vi "Pop-up wait prompt + events block.vi"(6 "Is Dialog?":enum16{"Normal", "Dialog Box"}(ring), 8 "error in (no error)":errorcluster, 9 "Prompt Text":string, 11 "Control":enum16{"Open", "Close", "Status", "No Change"}(ring)) -> (0 "error out":errorcluster)   [LabVIEW 2013]
doc: "If there is no error in, this vi will either open or close the calling panel which displays a prompt to wait. The input control determines whether the panel is opened or closed. Typically called before intensive processing with control=open and after with control = close.\n\nClose action ignores error in."
uses:
  GUI.lvlib
  Timing/Timing Lib.lvlib
panel:
  out "Prompt":string
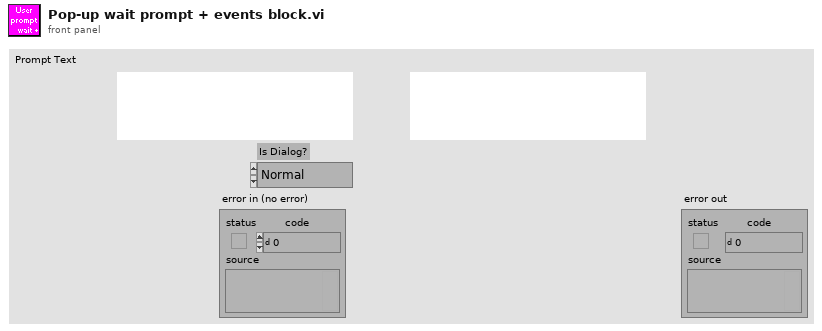
[diagram p1: front panel]
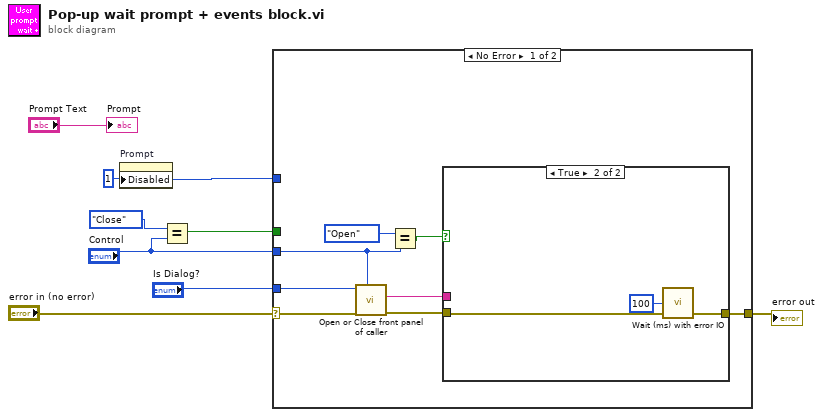
[diagram p0: block diagram]
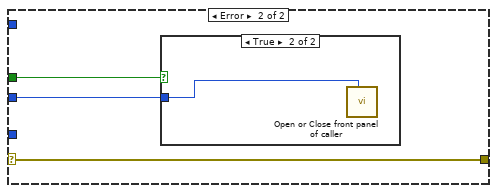
[diagram p3: hidden frame]
diagram:
  w4 = u8 1 ("Write Attribute")
  n1 = property on="Prompt" class="Str"("Disabled"=w4) -> ()  [unwired: 2 in, 2 out]
  n2 = Equal?(x=enum16{"Open", "Close", "Status", "No Change"}."Close", y="Control") -> (x = y?=w6:bool)
  n3 = case shown="No Error" "error in (no error)" {
    selector: "error in (no error)" -> [w11 w21]
    tunnel: [w12 w21] -> w8
    tunnel: w6 -> [_ w23]
    tunnel: "Control" -> [w16 w22]
    tunnel: w4 -> [_ _]
    tunnel: "Is Dialog?" -> [w9 _]
    frame No Error {
      n4 = call "Open or Close front panel of caller.vi"("Control"=w16, "error in (no error)"=w11, "Is Dialog?"=w9) -> ("error out"=w13:errorcluster, "Calling VI"=w10:string)  [unwired: 1 in, 4 out]
      n5 = Equal?(x=enum16{"Open", "Close", "Status", "No Change"}."Open", y=w16) -> (x = y?=w14:bool)
      n6 = case shown="True" w14 {
        tunnel: w13 -> [w17 w18]
        tunnel: [w17 w20] -> w12
        tunnel: w10 -> [_ _]
        frame False {
        }
        frame True {
          n7 = call "Wait (ms) with error IO.vi"("error in (no error)"=w18, "milliseconds to wait"=u32 100) -> ("error out"=w20:errorcluster)  [unwired: 3 out]
        }
      }
    }
    frame Error {
      n8 = case shown="True" w23 {
        tunnel: w22 -> [_ w24]
        frame False {
        }
        frame True {
          n9 = call "Open or Close front panel of caller.vi"("Control"=w24) -> ()  [unwired: 3 in, 6 out]
        }
      }
    }
  }
  "error out" <- w8
  "Prompt" <- "Prompt Text"
